vi "BatchTest TimePeriod.vi"(5 "Initialize?":bool, 9 "error in (no error)":errorcluster) -> (6 "Time(mS)":u32, 10 "error out":errorcluster)   [LabVIEW 2013]
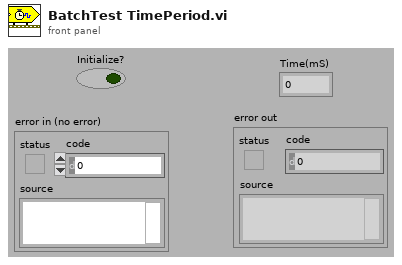
[diagram p1: front panel]
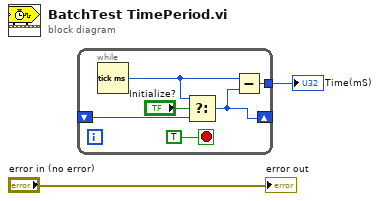
[diagram p0: block diagram]
diagram:
  n1 = while {
    shift-right: [w4] -> _
    shift-left: _ -> [w5]
    tunnel: [w3] -> w2
    stop <- TRUE stop-if-true
    n2 = Tick Count (ms)() -> (millisecond timer value=w6:u32)
    n3 = Select(t=w6, s="Initialize?", f=w5) -> (s? t:f=w4:u32)
    n4 = Subtract(x=w6, y=w4) -> (x-y=w3:u32)
  }
  "Time(mS)" <- w2
  "error out" <- "error in (no error)"
